vi "Update Point Data.vi"(8 "error in":errorcluster, 9 "Data":variant, 10 "Task-Point Ident":string, 11 "ISeries UI Actor in":refnum<class "ISeries UI Actor.lvclass">) -> (0 "error out":errorcluster, 3 "ISeries UI Actor out":refnum<class "ISeries UI Actor.lvclass">)   [LabVIEW 2024, in "ISeries UI Actor.lvlib" / "ISeries UI Actor.lvclass"]
uses:
  ISeries UI Actor.lvclass
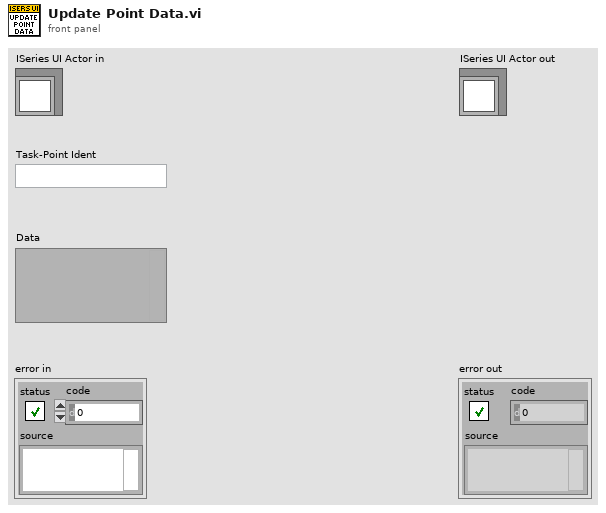
[diagram p1: front panel]
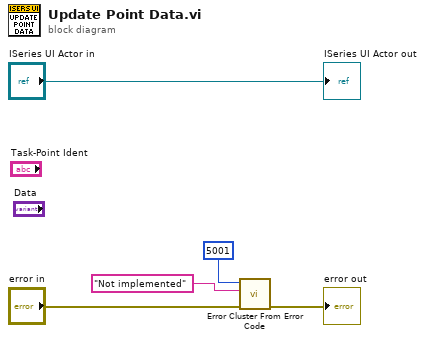
[diagram p0: block diagram]
diagram:
  n1 = call <vilib>:"Error Cluster From Error Code.vi"("error in (no error)"="error in", "error message (\"\")"="Not implemented" ("error message (\"\")"), "error code (0)"=5001) -> ("error out"=→"error out":errorcluster)  [unwired: 6 in]
  "ISeries UI Actor out" <- "ISeries UI Actor in"
